vi "保存CSV文件头.vi"(6 "单位":string, 7 "当前时间":timestamp, 8 "数据存储路径":path, 9 "采样率":u32, 10 "实际备注数组":string[](array[string]), 11 "error in (no error)":errorcluster caption="错误输入（无错误）") -> (0 "实际存储路径":path caption="新建文件路径（取消时为非法路径）", 3 "error out":errorcluster caption="错误输出")   [LabVIEW 2016]
uses:
  <vilib>/Utility/file.llb/Write To Spreadsheet File (string).vi
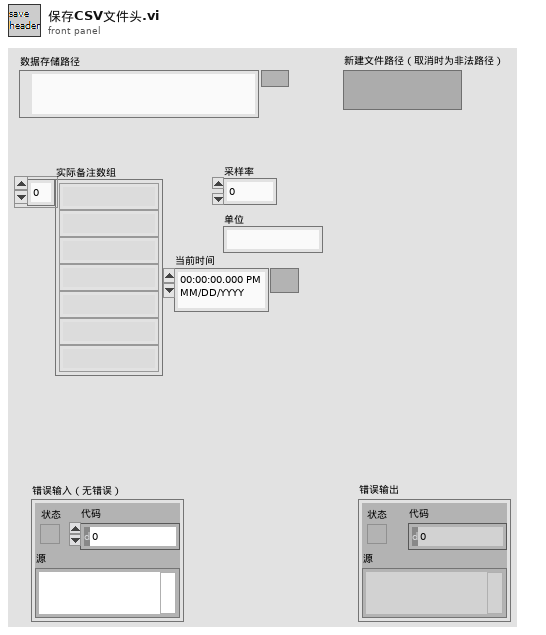
[diagram p1: front panel]
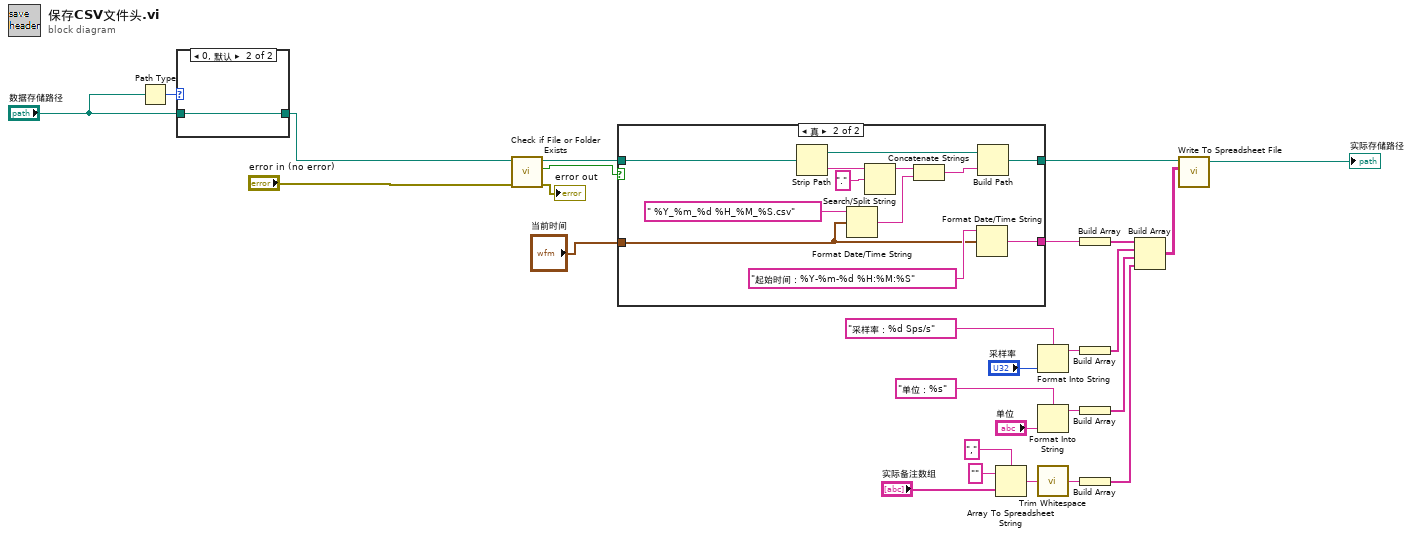
[diagram p0: block diagram]
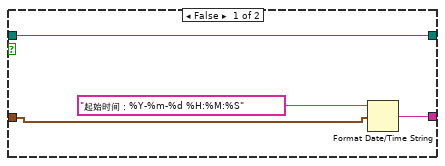
[diagram p2: hidden frame]
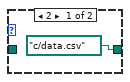
[diagram p3: hidden frame]
diagram:
  n1 = Path Type(1:"数据存储路径") -> (0:w27:i16)
  n2 = case shown="0, 默认" w27 {
    tunnel: "数据存储路径" -> [_ w29]
    tunnel: [path "c:/data.csv" w29] -> w23
    frame 2 {
    }
    frame 0, Default {
    }
  }
  n3 = call <vilib>:"Check if File or Folder Exists.vi"("error in (no error)"="error in (no error)", "path"=w23) -> ("error out"=→"error out":errorcluster, "file or folder exists?"=w21:bool, "dup path"=w22:path)  [unwired: 7 in]
  n4 = case shown="真" w21 {
    tunnel: w22 -> [w33 w45]
    tunnel: [w33 w37] -> w1
    tunnel: [w31 w35] -> w20
    tunnel: "当前时间" -> [w30 w34]
    frame False {
      n5 = Format Date/Time String(time format string (%c)="起始时间：%Y-%m-%d %H:%M:%S" ("时间格式字符串(%c)"), seconds (now)=w30) -> (date/time string=w31:string)  [unwired: 1 in]
    }
    frame True {
      n6 = Strip Path(path=w45) -> (stripped path=w39:path, name=w42:string)
      n7 = Format Date/Time String(time format string (%c)=" %Y_%m_%d %H_%M_%S.csv" ("时间格式字符串(%c)"), seconds (now)=w34) -> (date/time string=w43:string)  [unwired: 1 in]
      n8 = Search/Split String(string=w42, search string/char (-)="." ("搜索字符串/字符(-)")) -> (substring before match=w40:string)  [unwired: 1 in, 2 out]
      n9 = Concatenate Strings(w40, w43) -> (w38:string)
      n10 = Format Date/Time String(time format string (%c)="起始时间：%Y-%m-%d %H:%M:%S" ("时间格式字符串(%c)"), seconds (now)=w34) -> (date/time string=w35:string)  [unwired: 1 in]
      n11 = Build Path(base path=w39, name or relative path=w38) -> (appended path=w37:path)
    }
  }
  n12 = Array To Spreadsheet String(delimiter (Tab)="," ("分隔符(Tab)"), array="实际备注数组", 3:"" ("格式字符串")) -> (spreadsheet string=w13:string)
  n13 = Format Into String(format string="采样率：%d Sps/s" ("格式字符串"), "采样率") -> (resulting string=w9:string)  [unwired: 2 in, 1 out]
  n14 = Format Into String(format string="单位：%s" ("格式字符串"), "单位") -> (resulting string=w6:string)  [unwired: 2 in, 1 out]
  n15 = call <vilib>:"Trim Whitespace.vi"("string"=w13) -> ("trimmed string"=w12:string)  [unwired: 1 in]
  n16 = Build Array(w20) -> (w19:string[])
  n17 = Build Array(w9) -> (w8:string[])
  n18 = Build Array(w6) -> (w5:string[])
  n19 = Build Array(w12) -> (w4:string[])
  n20 = Build Array(w19, w8, w5, w4) -> (w18:string[][])
  n21 = call-poly <vilib>:"Write To Spreadsheet File.vi"("2D data"=w18, "file path (dialog if empty)"=w1) -> ("new file path (Not A Path if cancelled)"=→"实际存储路径":path)  [unwired: 6 in]
